vi "ArmGoalJointAngleCalculations.vi"(1 "Goal End Effector Position":cluster{dbl, dbl, dbl}, 2 "Intial Joint Angle Guesses (deg)":cluster{dbl, dbl, dbl}) -> (0 "Goal Joint Angles (deg)":cluster{dbl, dbl, dbl})   [LabVIEW 2020]
doc: "Calculates goal joint angles for the shoulder, elbow, and wrist based on goal (X,Z,pitch) coordinates. This VI uses a modified version of NI's Inverse Kinematics solver."
uses:
  4e757515-8708-4b3b-af8e-308136e6e1b4.vi
  b0bf9f40-873f-4d67-88ca-c4ea0c875f2e.vi
  <vilib>/robotics/Kinematics/RotateX.vi
  <vilib>/robotics/Kinematics/RotateY.vi
  <vilib>/robotics/Kinematics/RotateZ.vi
  <vilib>/Analysis/baseanly.llb/A x B.vi
  <vilib>/Analysis/baseanly.llb/Real A x B.vi
  GlobalArm.vi
  GlobalDriverStationData.vi
  <vilib>/Analysis/Matrix/Comparison/Not Equal/Not Equal.vi
  <vilib>/Analysis/Matrix/Comparison/Not Equal/Not Equal - RM,RM.vi
  <vilib>/robotics/Kinematics/NI_Kinematics.lvlib
panel:
  out "IK Error":errorcluster
  out "Steps Taken":i32
  # "Shoulder (deg)"
  # "Shoulder (deg)"
  # "Elbow (deg)"
  # "Elbow (deg)"
  # "Wrist (deg)"
  # "Wrist (deg)"
  # "Pitch (deg)"
  # "X (in)"
  # "Z (in)"
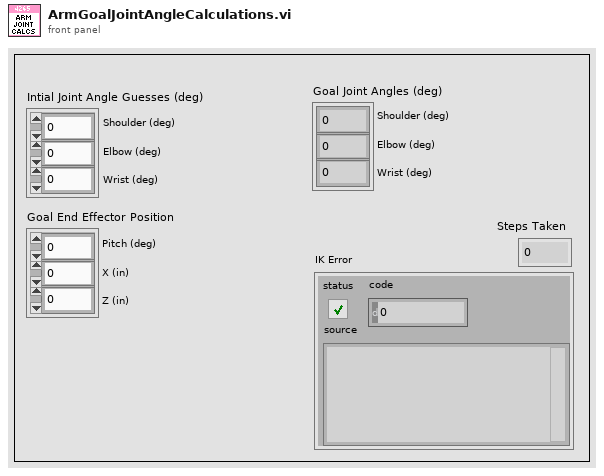
[diagram p1: front panel]
types:
  T1 = typedef "NI_Matrix.lvlib/RealMatrix.ctl" = dbl[][]
  T2 = cluster{"element":dbl, "element":dbl, "element":dbl}
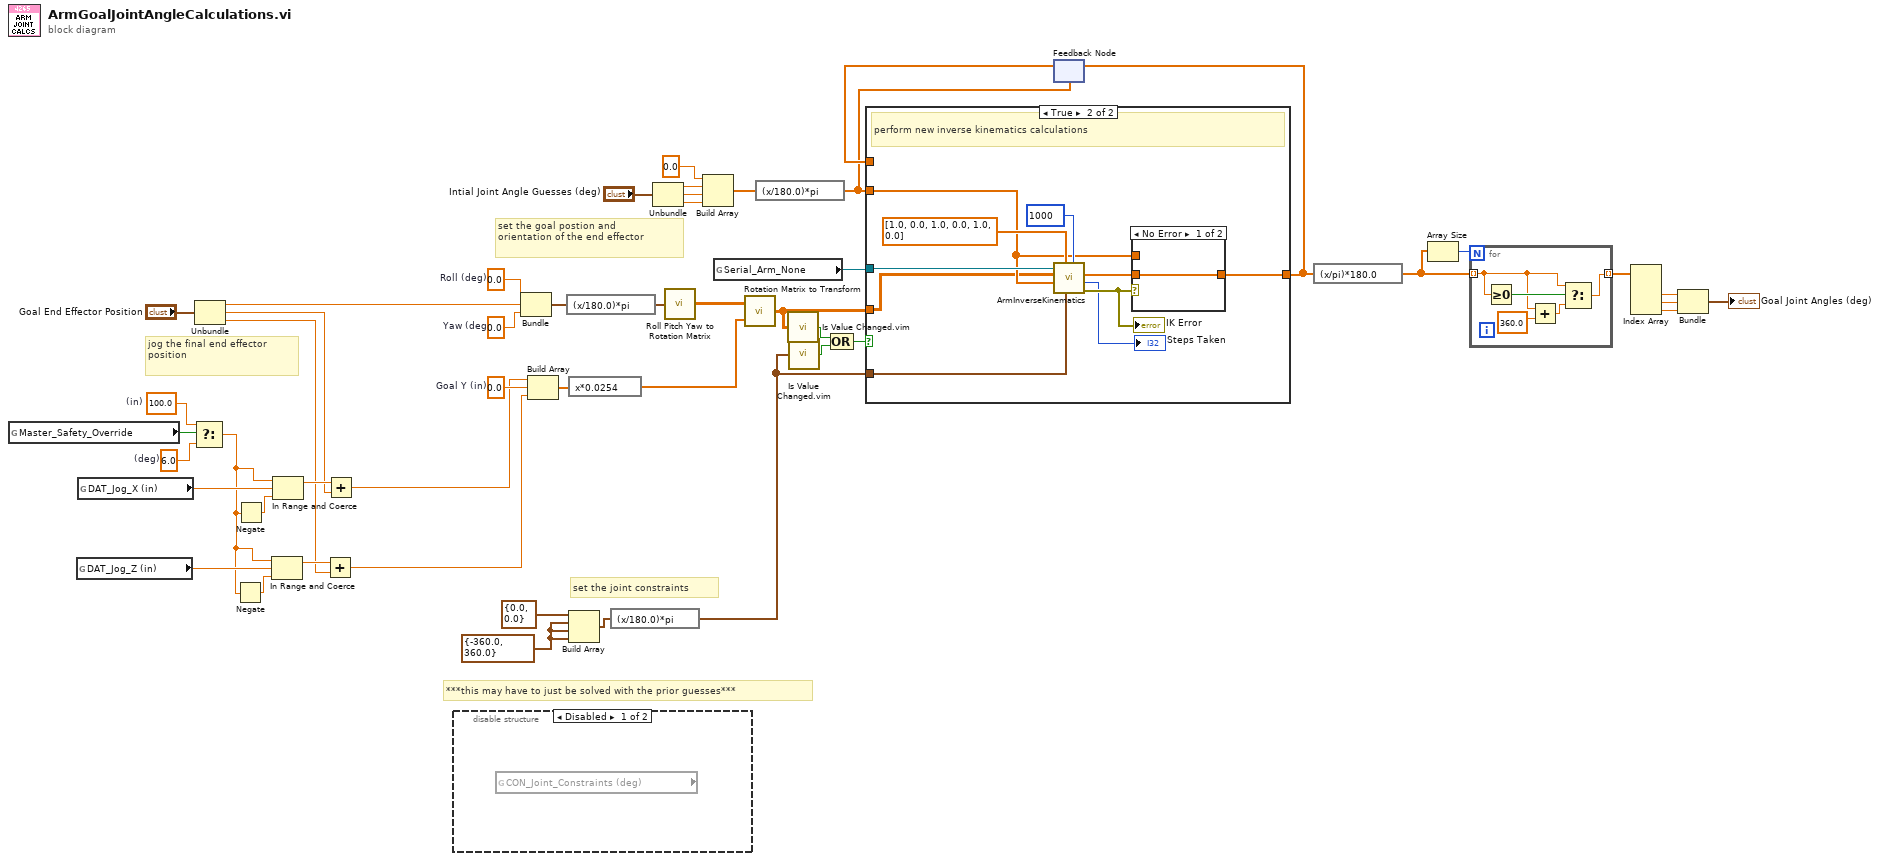
[diagram p0: block diagram]
diagram:
  w5 = cluster{dbl, dbl} {-360.0, 360.0}
  w10 = 100.0  # (in)
  w11 = 6.0  # (deg)
  w38 = 0.0  # Yaw (deg
  w39 = 0.0  # Roll (deg)
  w41 = 0.0  # Goal Y (in)
  # "***this may have to just be solved with the prior guesses***"
  # "jog the final end effector\nposition"
  # "set the joint constraints"
  # "set the goal postion and\norientation of the end effector"
  n1 = global read "GlobalDriverStationData.vi" "Master_Safety_Override"() -> (w12:bool)
  n2 = global read "GlobalArm.vi" "DAT_Jog_Z (in)"() -> (w17:dbl)
  n3 = global read "GlobalArm.vi" "DAT_Jog_X (in)"() -> (w22:dbl)
  n4 = Select(t=w10, s=w12, f=w11) -> (s? t:f=w9:dbl)
  n5 = Unbundle("Goal End Effector Position") -> (w29:dbl, w19:dbl, w14:dbl)
  n6 = Negate(x=w9) -> (-x=w16:dbl)
  n7 = Negate(x=w9) -> (-x=w21:dbl)
  n8 = In Range and Coerce(upper limit=w9, x=w17, lower limit=w16) -> (coerced(x)=w15:dbl)  [unwired: 1 out]
  n9 = In Range and Coerce(upper limit=w9, x=w22, lower limit=w21) -> (coerced(x)=w20:dbl)  [unwired: 1 out]
  n10 = Add(x=w15, y=w14) -> (x+y=w13:dbl)
  n11 = Add(x=w20, y=w19) -> (x+y=w18:dbl)
  n12 = disable-structure shown="Disabled" {
    frame Disabled {
      n13 = global read "GlobalArm.vi" "CON_Joint_Constraints (deg)"() -> ()  [unwired: 1 out]
    }
    frame Enabled {
    }
  }
  n14 = Bundle("Roll (deg)"=w39, w29, "Yaw (deg"=w38) -> (w40:cluster{"Roll (deg)":dbl, dbl, "Yaw (deg":dbl})  [unwired: 1 in]
  n15 = Build Array(w18, w41, w13) -> (w46:dbl[])
  n16 = expression code="(x/180.0)*pi" ("degrees to radians")(w40) -> (w45:cluster{"Roll (deg)":dbl, dbl, "Yaw (deg":dbl})
  n17 = expression code="x*0.0254" ("degrees to radians")(w46) -> (w42:dbl[])
  n18 = Build Array(cluster{dbl, dbl} {0.0, 0.0}, w5, w5, w5) -> (w33:cluster{dbl, dbl}[])
  n19 = expression code="(x/180.0)*pi" ("degrees to radians")(w33) -> (w32:cluster{dbl, dbl}[])
  n20 = Unbundle("Intial Joint Angle Guesses (deg)") -> (w23:dbl, w24:dbl, w25:dbl)
  n21 = call <vilib>:"Roll Pitch Yaw to Rotation Matrix.vi"("angles"=w45) -> ("rotation matrix"=w44:T1)
  n22 = Build Array(0.0 ("element"), w23, w24, w25) -> (w26:dbl[])
  n23 = global read "GlobalArm.vi" "Serial_Arm_None"() -> (w37:refnum<class "NI_Robotics_Serial Robot Arm.lvclass">)
  n24 = call <vilib>:"Rotation Matrix to Transform.vi"("translation vector"=w42, "rotation matrix"=w44) -> ("transform"=w43:T1)
  n25 = expression code="(x/180.0)*pi" ("degrees to radians")(w26) -> (w35:dbl[])
  n26 = call "Is Value Changed.vim"("value"=w43) -> ("changed or first call?"=w48:bool)
  n27 = call "Is Value Changed.vim"("value"=w32) -> ("changed or first call?"=w49:bool)
  n28 = Compound Arithmetic op=OR(w48, w49) -> (w47:bool)
  n29 = feedback #1(w35) -> (w36:dbl[])
  n30 = case shown="True" w47 {
    tunnel: [w50 w58] -> w34
    tunnel: w37 -> [_ w56]
    tunnel: w35 -> [_ w54]
    tunnel: w32 -> [_ w53]
    tunnel: w43 -> [_ w52]
    tunnel: w36 -> [w50 _]
    frame False {
      # "the end effector goal postion has not changed"
    }
    frame True {
      # "perform new inverse kinematics calculations"
      n31 = call "ArmInverseKinematics.vi"("max steps"=1000, "joint constraints"=w53, "mask"=dbl[] [1.0, 0.0, 1.0, 0.0, 1.0, 0.0], "current joint positions"=w54, "end effector transform"=w52, "serial arm in"=w56) -> ("error out"=w57:errorcluster, "steps taken"=→"Steps Taken":i32, "joint positions"=w59:dbl[])  [unwired: 2 in, 1 out]
      "IK Error" <- w57
      n32 = case shown="No Error" w57 {
        tunnel: w59 -> [w61 _]
        tunnel: [w61 w62] -> w58
        tunnel: w54 -> [_ w62]
        frame No Error {
        }
        frame Error {
        }
      }
    }
  }
  n33 = feedback-in #1(w34) -> ()
  n34 = expression code="(x/pi)*180.0" ("radians to degrees")(w34) -> (w2:dbl[])
  n35 = Array Size(array=w2) -> (size(s)=w1:i32)
  n36 = for {
    N: w1 -> [_]
    tunnel: w2 -> [w65] mode=indexing
    tunnel: [w66] -> w3 mode=indexing
    n37 = Greater Or Equal To 0?(x=w65) -> (x >= 0?=w67:bool)
    n38 = Add(x=w65, y=360.0) -> (x+y=w64:dbl)
    n39 = Select(t=w65, s=w67, f=w64) -> (s? t:f=w66:dbl)
  }
  n40 = Index Array(array=w3) -> (element #2=w6:dbl, element #3=w7:dbl, element #4=w8:dbl)  [unwired: 4 in, 1 out]
  n41 = Bundle("element"=w6, "element"=w7, "element"=w8) -> (→"Goal Joint Angles (deg)":T2)  [unwired: 1 in]
